vi "Initialize Hardware.vi"(8 "error in (no error)":errorcluster, 11 "DemoMicrosope in":refnum<class "DemoMicrosope.lvclass">) -> (0 "error out":errorcluster, 3 "DemoMicrosope out":refnum<class "DemoMicrosope.lvclass">)   [LabVIEW 2020]
uses:
  DemoMicrosope.lvclass
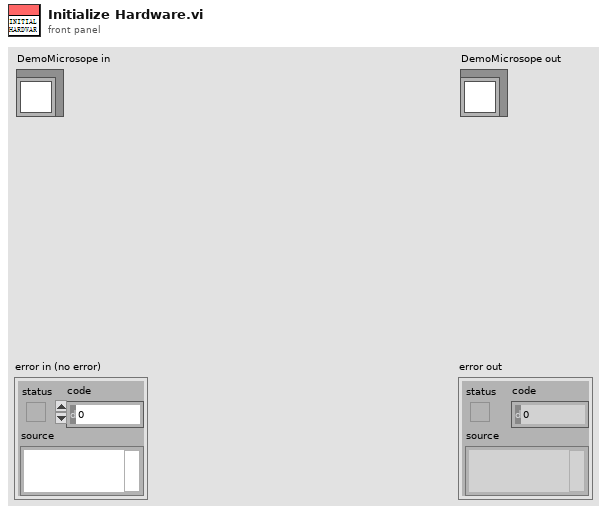
[diagram p1: front panel]
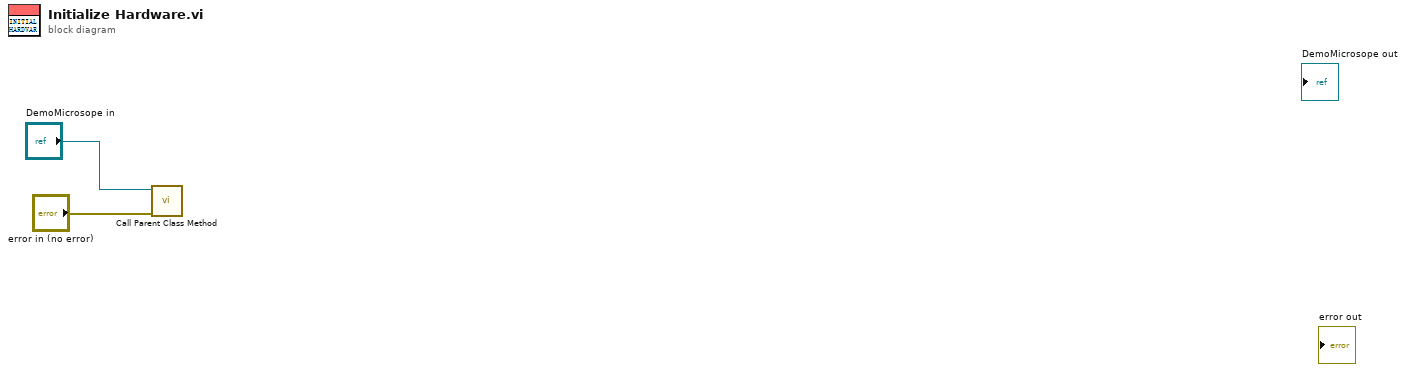
[diagram p0: block diagram]
diagram:
  n1 = call-parent "Call Parent Class Method"("error in (no error)"="error in (no error)", "Microscope in"="DemoMicrosope in") -> ("error out"=w3:errorcluster, "Microscope out"=w4:refnum<class "DemoMicrosope.lvclass">)  [unwired: 8 in]
